vi "Stop Dispatcher.vi"(11 "error in":errorcluster) -> (15 "error out":errorcluster)   [LabVIEW 2009, in "AMC.lvlib"]
doc: "Terminates the Dispatcher process."
uses:
  AMC.lvlib
  Globals.vi
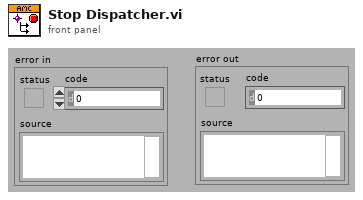
[diagram p1: front panel]
types:
  T1 = enum32{"Bad", "Idle", "Run top level", "Running"}
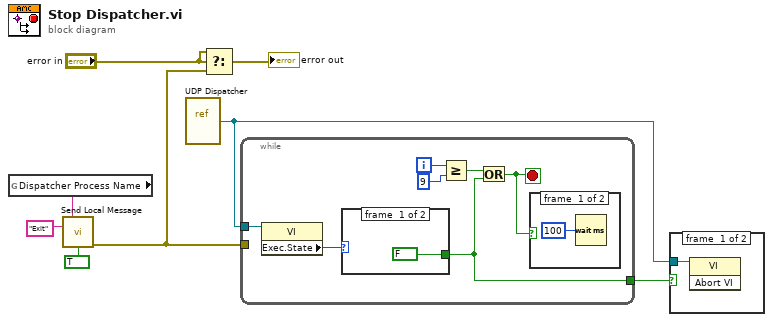
[diagram p0: block diagram]
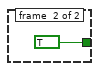
[diagram p4: hidden frame]
diagram:
  n1 = global read "Globals.vi" "Dispatcher Process Name"() -> (w5:string)
  n2 = call "Send Local Message.vi"("receiver process (\"\" - local)"=w5, "message name"="Exit" ("Name"), "priority message (F)"=TRUE) -> ("error out"=w3:errorcluster)  [unwired: 10 in, 2 out]
  n3 = vi-ref "UDP Dispatcher.vi"() -> (w7:refnum<vi>)
  n4 = Select(t="error in", s="error in", f=w3) -> (s? t:f=→"error out":errorcluster)
  n5 = while {
    tunnel: w7 -> [w15]
    tunnel: [w9] -> w8
    tunnel: w3 -> [_]
    i -> [w13]
    stop <- w10 stop-if-true
    n6 = property class="VI"(reference=w15) -> ("Exec.State"=w14:T1)  [unwired: 1 in, 2 out]
    n7 = case shown="\"Run top level\"" w14 {
      tunnel: [FALSE TRUE] -> w9
      frame #0 {
      }
      frame #1 {
      }
    }
    n8 = Greater Or Equal?(x=w13, y=9) -> (x >= y?=w11:bool)
    n9 = Or(x=w11, y=w9) -> (x .or. y?=w10:bool)
    n10 = case shown="False" w10 {
      frame #0 {
        n11 = Wait (ms)(milliseconds to wait=u32 100) -> ()  [unwired: 1 out]
      }
      frame #1 {
      }
    }
  }
  n12 = case shown="False" w8 {
    tunnel: w7 -> [w19 _]
    frame #0 {
      n13 = invoke class="VI" method="Abort VI"(reference=w19) -> ()  [unwired: 2 in, 3 out]
    }
    frame #1 {
    }
  }
